vi "loadSRMFiles.vi"(7 "working directory":path=path "c:/temp", 11 "folder":string="192.168.1.13\\equ-summary\\hexa\\FLST08") -> ()   [LabVIEW 2012]
panel:
  out "Output":string
  out "OK":bool
  out "concatenated string":string
  out "error out":errorcluster
  in  "error in (no error)":errorcluster
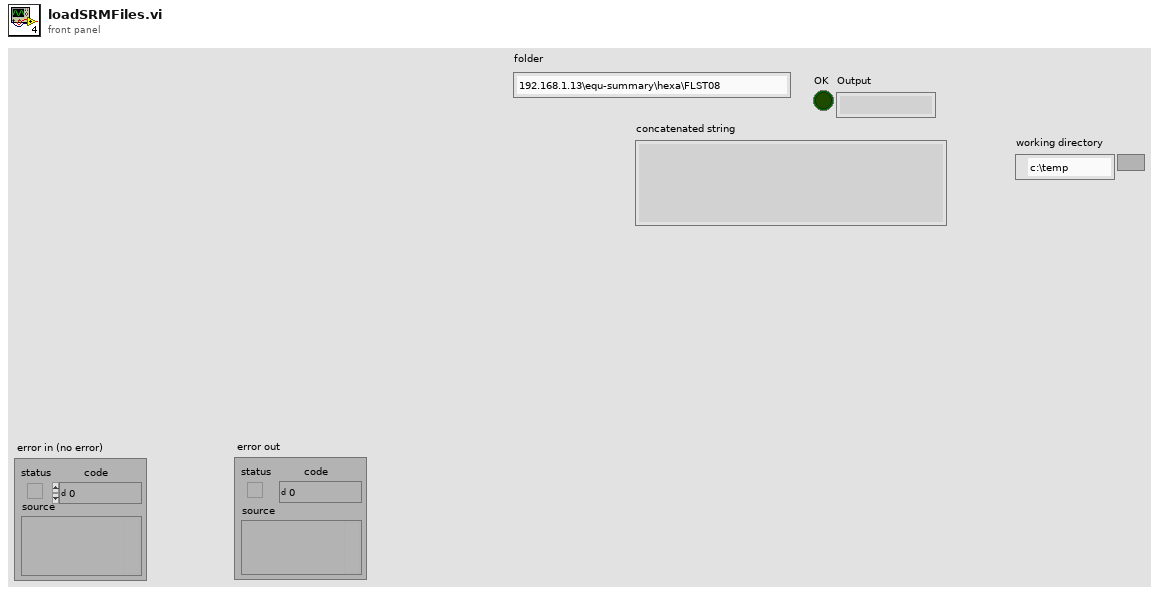
[diagram p1: front panel]
types:
  T1 = enum16{"open", "replace", "create", "open or create", "replace or create", "replace or create with confirmation"}
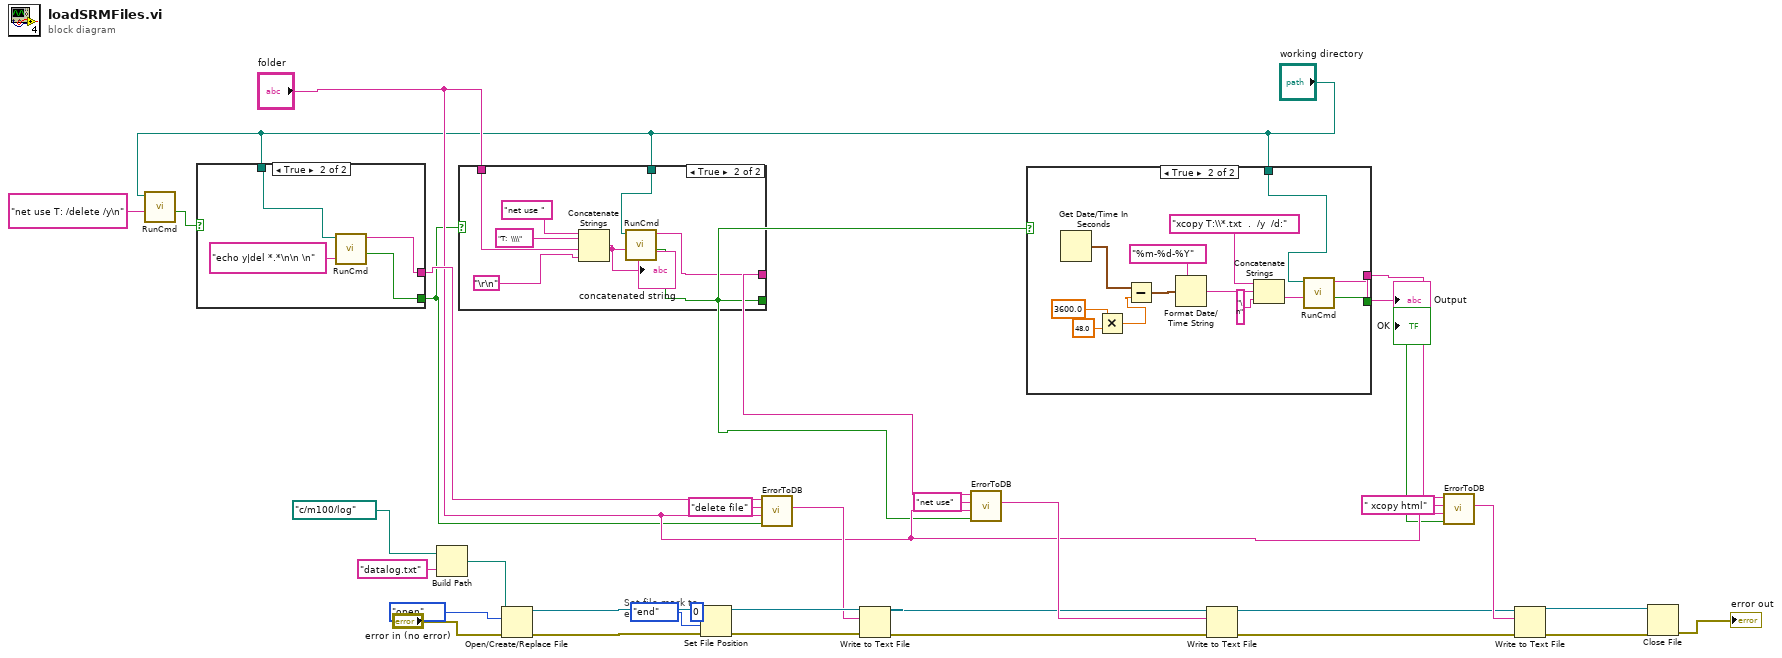
[diagram p0: block diagram]
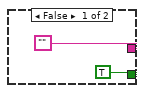
[diagram p2: hidden frame]
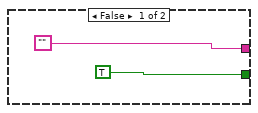
[diagram p3: hidden frame]
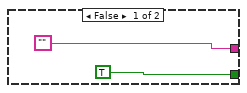
[diagram p4: hidden frame]
diagram:
  # "Set file mark to\nend of file"
  n1 = call "RunCmd.vi"("Cmd String"="net use T: /delete /y\n" ("string"), "working directory"="working directory") -> ("OK"=w20:bool)  [unwired: 8 in, 1 out]
  n2 = case shown="True" w20 {
    tunnel: [TRUE w38] -> w8
    tunnel: ["" w37] -> w15
    tunnel: "working directory" -> [_ w40]
    frame False {
    }
    frame True {
      n3 = call "RunCmd.vi"("Cmd String"="echo y|del *.*\n\n \n" ("standard input"), "working directory"=w40) -> ("OK"=w38:bool, "Output"=w37:string)  [unwired: 8 in]
    }
  }
  n4 = Build Path(base path=path "c:/m100/log", name or relative path="datalog.txt") -> (appended path=w26:path)
  n5 = case shown="True" w8 {
    tunnel: [TRUE w43] -> w1
    tunnel: ["" w44] -> w23
    tunnel: "folder" -> [_ w46]
    tunnel: "working directory" -> [_ w45]
    frame False {
    }
    frame True {
      n6 = Concatenate Strings("net use " ("string"), "T:  \\\\" ("string"), w46, "\r\n") -> (w50:string)
      "concatenated string" <- w50
      n7 = call "RunCmd.vi"("Cmd String"=w50, "working directory"=w45) -> ("OK"=w43:bool, "Output"=w44:string)  [unwired: 8 in]
    }
  }
  n8 = Open/Create/Replace File(file path (use dialog)=w26, error in="error in (no error)", operation (0:open)=T1."open") -> (refnum out=w31:refnum<file>, error out=w30:errorcluster)  [unwired: 3 in, 1 out]
  n9 = Set File Position(offset (in bytes) (0)=i64 0, refnum=w31, from (0:start)=enum16{"start", "end", "current"}."end", error in=w30) -> (refnum out=w19:refnum<file>, error out=w18:errorcluster)
  n10 = call "ErrorToDB.vi"("Error"=w8, "Folder"="folder", "Command"="delete file", "Error Message"=w15) -> ("LogData"=w14:string)  [unwired: 7 in]
  n11 = Write to Text File(file (use dialog)=w19, text=w14, error in=w18) -> (refnum out=w17:refnum<file>, error out=w16:errorcluster)  [unwired: 1 in, 1 out]
  n12 = call "ErrorToDB.vi"("Error"=w1, "Folder"="folder", "Command"="net use", "Error Message"=w23) -> ("LogData"=w25:string)  [unwired: 7 in]
  n13 = case shown="True" w1 {
    tunnel: [TRUE w53] -> w9
    tunnel: ["" w54] -> w22
    tunnel: "working directory" -> [_ w65]
    frame False {
    }
    frame True {
      n14 = Get Date/Time In Seconds() -> (seconds since 1Jan1904=w55:timestamp)
      n15 = Multiply(x=3600.0, y=48.0) -> (x*y=w57:dbl)
      n16 = Subtract(x=w55, y=w57) -> (x-y=w58:timestamp)
      n17 = Format Date/Time String(time format string (%c)="%m-%d-%Y", seconds (now)=w58) -> (date/time string=w61:string)  [unwired: 1 in]
      n18 = Concatenate Strings("xcopy T:\\*.txt  .  /y  /d:" ("string"), w61, "\n" ("string")) -> (w64:string)
      n19 = call "RunCmd.vi"("Cmd String"=w64, "working directory"=w65) -> ("OK"=w53:bool, "Output"=w54:string)  [unwired: 8 in]
    }
  }
  "OK" <- w9
  "Output" <- w22
  n20 = Write to Text File(file (use dialog)=w17, text=w25, error in=w16) -> (refnum out=w3:refnum<file>, error out=w2:errorcluster)  [unwired: 1 in, 1 out]
  n21 = call "ErrorToDB.vi"("Error"=w9, "Folder"="folder", "Command"=" xcopy html", "Error Message"=w22) -> ("LogData"=w21:string)  [unwired: 7 in]
  n22 = Write to Text File(file (use dialog)=w3, text=w21, error in=w2) -> (refnum out=w6:refnum<file>, error out=w5:errorcluster)  [unwired: 1 in, 1 out]
  n23 = Close File(refnum=w6, error in=w5) -> (error out=→"error out":errorcluster)  [unwired: 1 out]
